vi "Regler Pumpe.vi"(7 "Index":i32, 8 "Fehler":errorcluster caption="Fehler (Eingang)") -> (0 "Fehler (Ausgang)":errorcluster)   [LabVIEW 2020, in "Regler.lvlib" / "Druckregler.lvlib"]
uses:
  Druckregler.lvlib
  Aktionen Param. Druckregler.ctl
  Aktionen Interne Werte.ctl
  Verwaltung/FGV IN Aktionen.ctl
  Konfig-Dateien/FGV Betriebsdaten Aktionen.ctl
  Verwaltung/FGV OUT Aktionen.ctl
  Verwaltung/Verwaltung - cRIO.lvlib
  Konfig-Dateien/Konfig-Dateien.lvlib
  Regler.lvlib
  Aktion FGV Werte vorgeben.ctl
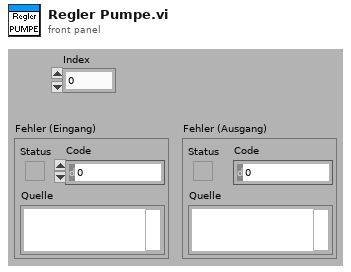
[diagram p1: front panel]
types:
  T1 = typedef "Verwaltung - cRIO.lvlib/FGV OUT Aktionen.ctl" = enum16{"lesen", "ANA OUT", "DO 0-31", "DO 32-47"}
  T2 = typedef "Konfig-Dateien.lvlib/FGV Betriebsdaten Aktionen.ctl" = enum16{"lesen", "Anlagengrenzw.", "PID Param.", "Sonstige", "Sensor Para."}
  T3 = typedef "Verwaltung - cRIO.lvlib/FGV IN Aktionen.ctl" = enum16{"lesen", "DI", "AI", "Fühler Br.", "TC", "Fühler Br. TC"}
  T4 = typedef "Regler.lvlib/Druckregler.lvlib/Aktionen Interne Werte.ctl" = enum16{"lesen", "FT-IR", "Ausgang", "Pumpe", "laden", "speichern", "Änderung?", "Druck Kalter Block", "Dichtheitstest"}
  T5 = typedef "Regler.lvlib/Druckregler.lvlib/Aktionen Param. Druckregler.ctl" = enum16{"lesen", "schreiben", "Regler FT-IR", "Regler Ausgang", "Regler Durchfluss", "Regler PMA", "Regler NDIR", "Regler Filterblock", "Regler Gaskühler", "Regler Kalter Block"}
  T6 = typedef "Anlagengrenzwerte.lvlib/Anlagen-Grenzwerte Anzeige.ctl" = cluster{"Eingangsdruck FT-IR:":T7, "Durchfluss FT-IR:":T7, "Durchfluss CalGas:":T7, "Druck Ausgang:":T7, "Druck Kalter Block:":T7, "Heizleitungen intern:":T7, "Heizleitung zu FT-IR:":T7, "Heizung Filterblock:":T7, "Heizung Pumpe:":T7, "Heizleitung Extern SP1:":T7, "Heizleitung Extern SP2:":T7, "FT-IR Heizung Messzelle:":T7, "Schaltschranktemperatur:":T7, "Gaskühler:":T7}
  T7 = typedef "Anlagengrenzwerte.lvlib/Anlagen-Parameter Anzeige.ctl" = cluster{"Sollwert":sgl, "Warn-Min":sgl, "Warn-Max":sgl, "Abschalt-Min":sgl, "Abschalt-Max":sgl, "Regler":u16}
  T8 = typedef "Verwaltung - cRIO.lvlib/Analog Eingaenge.ctl" = cluster{"AI0: Durchfluss FT-IR":sgl, "AI1: Druck Ausgang":sgl, "AI2: Umgebungsdruck":sgl, "AI3: Druck FT-IR":sgl, "AI4: Druck CalGas":sgl, "AI5: Reserve":sgl, "AI6: Reserve":sgl, "AI7: Reserve":sgl, "Rohwert Durchfluss FT-IR":sgl, "Rohwert Druck Ausgang":sgl, "Rohwert Umgebungsdruck":sgl, "Rohwert Druck FT-IR":sgl, "Rohwert Druck CalGas":sgl, "Rohwert AI5":sgl, "Rohwert AI6":sgl, "Rohwert AI7":sgl, "Rohwert Diffdruck mbar FTIR":sgl}
  T9 = typedef "Verwaltung - cRIO.lvlib/Digital Ausgaenge 32-63.ctl" = cluster{"O32: Messgaspumpe EIN":bool, "O33: (Umgebungsluftpumpe)":bool, "O34: (Kondensatpumpe GK)":bool, "O35: Klima/Lüfter EIN":bool, "O36: Versorgung Heizungen":bool, "O37: Versorgung Heizungen":bool, "O38: (Gaskühler EIN (Freigabe))":bool, "O39: Störung FAS LP":bool, "O40: (Heizung Filterblock)":bool, "O41: Heizung HL zu FT-IR":bool, "O42: Heizung HL Extern SP1":bool, "O43: Heizung HL Extern SP2":bool, "O44: Heizung Reserve":bool, "O45: Heizung Reserve":bool, "O46: Statusbeleuchtung grün":bool, "O47: Statusbeleuchtung rot":bool}
  T10 = typedef "Regler.lvlib/Aktion FGV Werte vorgeben.ctl" = enum16{"lesen", "P-Flow", "D-Filterblock"}
  T11 = cluster{"Numerisch":sgl, "Numerisch":sgl, "Numerisch":sgl, "Numerisch":sgl, "Numerisch":sgl}
  T12 = typedef "Regler.lvlib/Druckregler.lvlib/Regler Interne Werte.ctl" = cluster{"PV":sgl, "D-action":sgl, "Error":sgl, "I-action":sgl, "OUT":sgl}
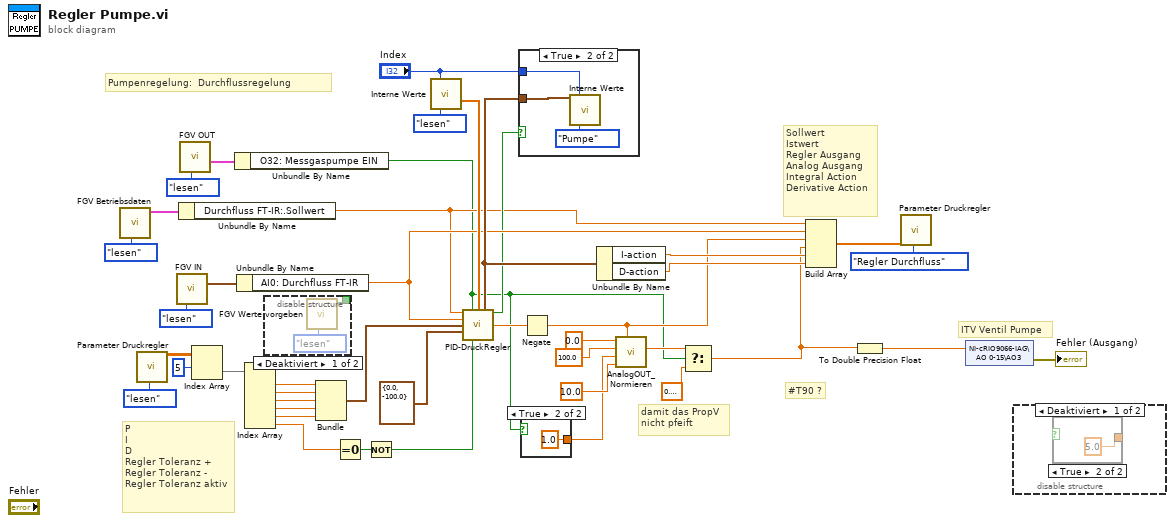
[diagram p0: block diagram]
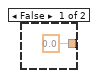
[diagram p3: hidden frame]
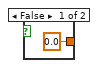
[diagram p6: hidden frame]
diagram:
  # "#T90 ?"
  # "damit das PropV\nnicht pfeift"
  # "Pumpenregelung:  Durchflussregelung"
  # "Sollwert\nIstwert\nRegler Ausgang\nAnalog Ausgang\nIntegral Action\nDerivative Action"
  # "P\nI\nD\nRegler Toleranz +\nRegler Toleranz -\nRegler Toleranz aktiv"
  # "ITV Ventil Pumpe"
  n1 = call "FGV Betriebsdaten.vi"("Aktionen"=FGV_Betriebsdaten_Aktionen."lesen") -> ("Anlagen-Grenzwerte"=w10:T6)  [unwired: 7 in, 3 out]
  n2 = call "Parameter Druckregler.vi"("Aktionen"=Aktionen_Param._Druckregler."lesen") -> ("Regleparameter"=w23:sgl[][])  [unwired: 10 in, 8 out]
  n3 = call "FGV IN.vi"("Aktion"=FGV_IN_Aktionen."lesen") -> ("Analog Eingänge"=w12:T8)  [unwired: 10 in, 4 out]
  n4 = Unbundle By Name(w10) -> ("Durchfluss FT-IR:.Sollwert"=w7:sgl)
  n5 = call "FGV OUT.vi"("Aktion"=FGV_OUT_Aktionen."lesen") -> ("DO 32-63"=w8:T9)  [unwired: 7 in, 3 out]
  n6 = Index Array(array=w23, index (row)=5 ("Index (Zeile)")) -> (element=w22:sgl[])  [unwired: 1 in]
  n7 = Unbundle By Name(w8) -> ("O32: Messgaspumpe EIN"=w1:bool)
  n8 = Unbundle By Name(w12) -> ("AI0: Durchfluss FT-IR"=w24:sgl)
  n9 = Index Array(array=w22) -> (element #1=w33:sgl, element #2=w32:sgl, element #3=w31:sgl, element #4=w30:sgl, element #5=w29:sgl, element #6=w20:sgl)  [unwired: 6 in]
  n10 = disable-structure shown="Deaktiviert" {
    disable-tunnel: [w44 _] -> _
    frame Disabled {
      n11 = call "FGV Werte vorgeben.vi"("Aktion"=Aktion_FGV_Werte_vorgeben."lesen") -> ("P-Flow"=w44:bool)  [unwired: 9 in, 1 out]
    }
    frame Enabled {
    }
  }
  n12 = Bundle("Numerisch"=w33, "Numerisch"=w32, "Numerisch"=w31, "Numerisch"=w30, "Numerisch"=w29) -> (w28:T11)  [unwired: 1 in]
  n13 = Equal To 0?(x=w20) -> (x = 0?=w27:bool)
  n14 = Not(x=w27) -> (.not. x?=w26:bool)
  n15 = call "Interne Werte.vi"("Index"="Index", "Aktionen Interne Werte"=Aktionen_Interne_Werte."lesen") -> ("Pumpe"=w39:sgl[])  [unwired: 7 in, 6 out]
  n16 = call "PID-DruckRegler.vi"("Sollwert"=w7, "Regler EIN"=w1, "Regler Interne Werte"=w39, "Istwert"=w24, "PID-Parameter"=w28, "output range"=cluster{"output high":sgl, "output low":sgl} {"output high"=0.0, "output low"=-100.0}, "Regler Toleranz verwenden?"=w26) -> ("Regler Interne Werte"=w38:T12, "Interne Werte speichern"=w16:bool, "Output"=w19:sgl)  [unwired: 6 in]
  n17 = case shown="True" w16 {
    tunnel: "Index" -> [_ w47]
    tunnel: w38 -> [_ w46]
    frame False {
    }
    frame True {
      n18 = call "Interne Werte.vi"("Regler Interne Werte"=w46, "Index"=w47, "Aktionen Interne Werte"=Aktionen_Interne_Werte."Pumpe") -> ()  [unwired: 6 in, 7 out]
    }
  }
  n19 = case shown="True" w1 {
    tunnel: [sgl 0.0 ("Untergrenze") sgl 1.0 ("Untergrenze")] -> w3
    frame False {
    }
    frame True {
    }
  }
  n20 = Negate(x=w19) -> (-x=w4:sgl)
  n21 = Unbundle By Name(w38) -> ("I-action"=w14:sgl, "D-action"=w15:sgl)
  n22 = call "AnalogOUT_Normieren.vi"("Analogwert"=w4, "Obergrenze"=sgl 10.0, "Untergrenze"=w3, "Max Analogwert"=sgl 100.0, "Min Analogwert"=sgl 0.0) -> ("Normierter Wert"=w6:sgl)  [unwired: 6 in]
  n23 = Select(t=w6, s=w1, f=sgl 0.2) -> (s? t:f=w2:sgl)
  n24 = Build Array(w7, w24, w4, w2, w14, w15) -> (w42:sgl[])
  n25 = To Double Precision Float(number=w2) -> (double precision float=w41:dbl)
  n26 = call "Parameter Druckregler.vi"("Werte Durchfluss"=w42, "Aktionen"=Aktionen_Param._Druckregler."Regler Durchfluss") -> ()  [unwired: 9 in, 9 out]
  n27 = shared-variable "NI-cRIO9066-IAG\\AO 0-15\\AO3"(w41) -> (error out=→"Fehler (Ausgang)":errorcluster)  [unwired: 1 in]
  n28 = disable-structure shown="Deaktiviert" {
    frame Disabled {
      n29 = case shown="True" {
        selector: _ -> [_ _]
        tunnel: [sgl 0.0 ("f") sgl 5.0 ("f")] -> _
        frame False {
        }
        frame True {
        }
      }
    }
    frame Enabled {
    }
  }
